vi "Acquire constant samples.vi"(0 "Instrument handle":refnum<k15>, 1 "Channel(s)":string, 2 "Cycles to acquire":u16=1 min=1, 3 "Samples/cycle":u32=1000 min=1, 4 "Frequency":dbl min=0.0 step=1000.0 format="%#_6p", 5 "error in (no error)":errorcluster) -> (14 "Instrument handle out":refnum<k15>, 15 "Waveform(s)":waveform(dbl)[](graph), 19 "error out":errorcluster)   [LabVIEW 2021]
uses:
  <instrlib>/niScope/Acquire/Fetch/niScope Multi Fetch WDT.vi
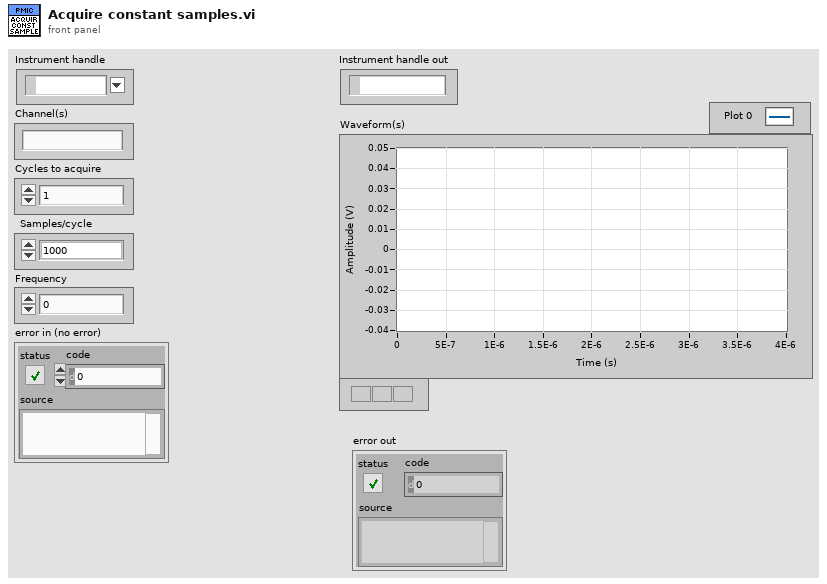
[diagram p1: front panel]
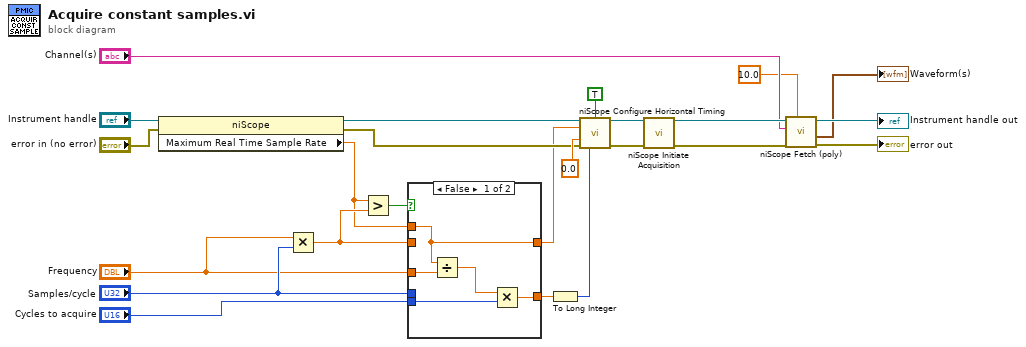
[diagram p0: block diagram]
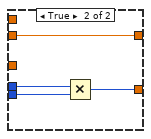
[diagram p2: hidden frame]
diagram:
  n1 = property class="niScope"(reference="Instrument handle", error in="error in (no error)") -> (reference out=w11:refnum<k15>, error out=w10:errorcluster, "Maximum Real Time Sample Rate"=w5:dbl)
  n2 = Multiply(x="Frequency", y="Samples/cycle") -> (x*y=w7:dbl)
  n3 = Greater?(x=w5, y=w7) -> (0:w9:bool)
  n4 = case shown="False" w9 {
    tunnel: "Cycles to acquire" -> [w25 w33]
    tunnel: "Samples/cycle" -> [_ w32]
    tunnel: [w27 w31] -> w4
    tunnel: "Frequency" -> [w29 _]
    tunnel: w7 -> [_ w30]
    tunnel: [w28 w30] -> w6
    tunnel: w5 -> [w28 _]
    frame False {
      n5 = Divide(x=w28, y=w29) -> (x/y=w26:dbl)
      n6 = Multiply(x=w26, y=w25) -> (x*y=w27:dbl)
    }
    frame True {
      n7 = Multiply(x=w32, y=w33) -> (x*y=w31:u32)
    }
  }
  n8 = To Long Integer(number=w4) -> (32bit integer=w3:i32)
  n9 = call <instrlib>:"niScope Configure Horizontal Timing.vi"("instrument handle"=w11, "enforce realtime"=TRUE, "min sample rate"=w6, "reference position"=0.0, "error in"=w10, "min record length"=w3) -> ("instrument handle out"=w22:refnum<k15>, "error out"=w21:errorcluster)  [unwired: 8 in]
  n10 = call <instrlib>:"niScope Initiate Acquisition.vi"("instrument handle"=w22, "error in"=w21) -> ("instrument handle out"=w20:refnum<k15>, "error out"=w19:errorcluster)  [unwired: 12 in]
  n11 = call-poly <instrlib>:"niScope Fetch (poly).vi"("timeout"=10.0, "error in"=w19, "channels"="Channel(s)", "instrument handle"=w20) -> ("error out"=→"error out":errorcluster, "wfm"=→"Waveform(s)":waveform(dbl)[], "instrument handle out"=→"Instrument handle out":refnum<k15>)  [unwired: 4 in, 1 out]
